vi "Local_Sense_Cmd_v1.vi"(7 "Control Board VISA":refnum<visa-resource-name>="ControlBoard", 8 "error in (no error)":errorcluster, 9 "Message IN":string, 10 "Relay Control":bool[](array[boolean]), 11 "LocalSenseRelayTask":refnum<k21>="BTS_LocalSenseRelays") -> (0 "error out":errorcluster, 1 "Message OUT":string, 2 "Voltage Array":dbl[](array[numeric]), 3 "LocalSenseRelayTaskOut":refnum<k21>)   [LabVIEW 2019]
uses:
  Ctls/ADC_Select_v1.ctl
  <vilib>/DAQmx/write.llb/DAQmx Write (Digital 1D Bool NChan 1Samp 1Line).vi
  <vilib>/DAQmx/miscellaneous.llb/DAQmx Fill In Error Info.vi
panel:
  out "Vline_ca":dbl
  out "Vline_ab":dbl
  out "Vline_bc":dbl
  out "Control Board OUT":refnum<visa-resource-name>
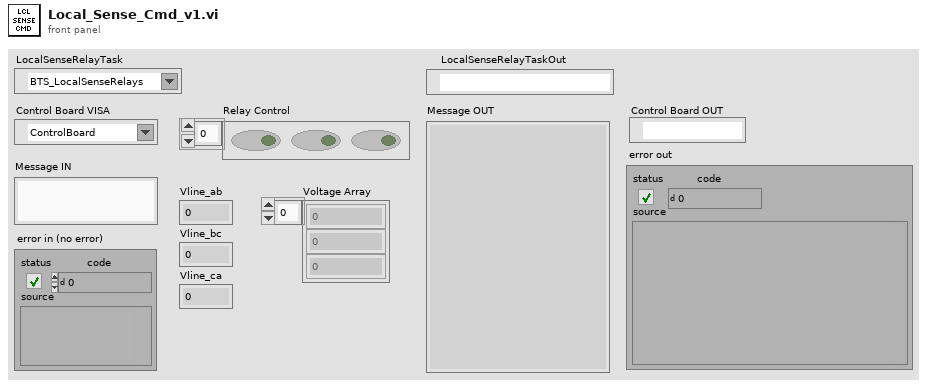
[diagram p1: front panel]
types:
  T1 = typedef "ADC_Select_v1.ctl" = enum16{"INVA_ISENSE_U", "INVA_ISENSE_V", "INVA_ISENSE_W", "INVA_UDC", "INVA_TEMP", "HB_TEMP", "AUXB_TEMP", "VLINE_AB", "VLINE_BC", "VLINE_CA", "VSENSE_POS_24V", "VSENSE_POS_5V", "VSENSE_NEG_15V", "INVB_ISENSE_U", "INV_B_ISENSEV", "INVB_ISENSE_W", "INVB_UDC", "INVB_TEMP", "AUXA_TEMP", "AUXC_TEMP", "VOUT_AB", "VOUT_BC", "VOUT_CA", "VSENSE_POS_15V", "VSENSE_POS_3P3V", "TEST_POINT"}
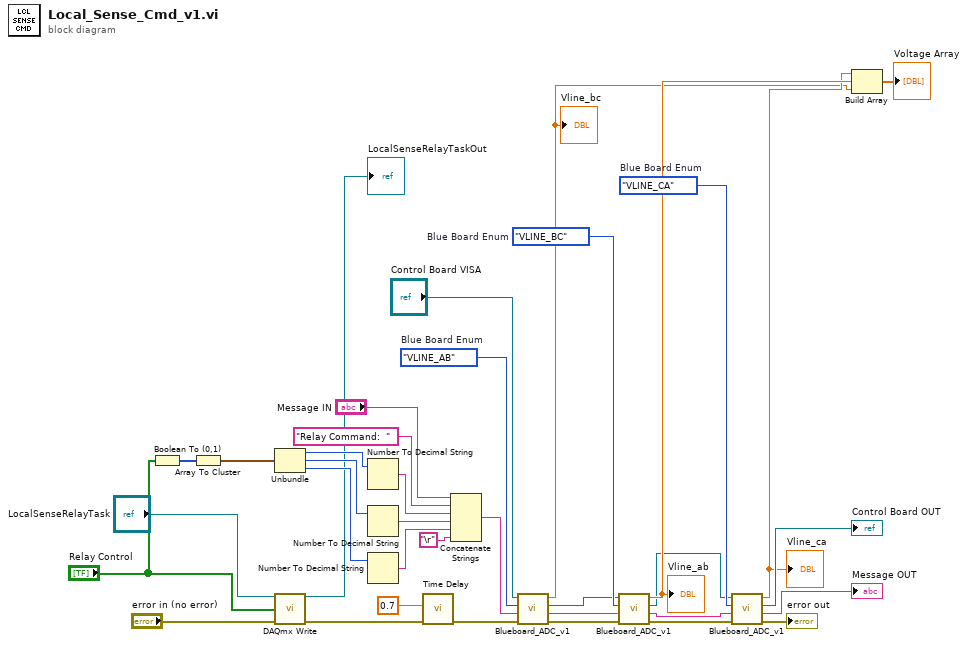
[diagram p0: block diagram]
diagram:
  w6 = ADC_Select_v1."VLINE_CA"  # Blue Board Enum
  w7 = ADC_Select_v1."VLINE_BC"  # Blue Board Enum
  w8 = ADC_Select_v1."VLINE_AB"  # Blue Board Enum
  n1 = Boolean To (0,1)(Boolean="Relay Control") -> (0, 1=w23:i16[])
  n2 = Array To Cluster(array=w23) -> (cluster=w22:cluster{"[0]":i16, "[1]":i16, "[2]":i16})
  n3 = Unbundle(w22) -> ("[0]"=w21:i16, "[1]"=w20:i16, "[2]"=w19:i16)
  n4 = call-poly <vilib>:"DAQmx Write.vi"("task/channels in"="LocalSenseRelayTask", "data"="Relay Control", "error in"="error in (no error)") -> ("task out"=→"LocalSenseRelayTaskOut":refnum<k21>, "error out"=w34:errorcluster)  [unwired: 10 in, 1 out]
  n5 = Number To Decimal String(number=w21) -> (decimal integer string=w16:string)  [unwired: 1 in]
  n6 = Number To Decimal String(number=w20) -> (decimal integer string=w17:string)  [unwired: 1 in]
  n7 = Number To Decimal String(number=w19) -> (decimal integer string=w18:string)  [unwired: 1 in]
  n8 = call "Time Delay"("error in (no error)"=w34, "Delay Time (s)"=0.7) -> ("error out"=w31:errorcluster)  [unwired: 9 in]
  n9 = Concatenate Strings("Message IN", "Relay Command:  ", w16, w17, w18, "\r") -> (w15:string)
  n10 = call "Blueboard_ADC_v1.vi"("error in (no error)"=w31, "Message IN"=w15, "Blue Board Enum"=w8, "ControlBoard VISA"="Control Board VISA") -> ("error out"=w36:errorcluster, "Message OUT"=w14:string, "VISA Refnum out"=w4:refnum<visa-resource-name>, "Result"=w28:dbl)  [unwired: 4 in]
  "Vline_bc" <- w28
  n11 = call "Blueboard_ADC_v1.vi"("error in (no error)"=w36, "Message IN"=w14, "Blue Board Enum"=w7, "ControlBoard VISA"=w4) -> ("error out"=w35:errorcluster, "Message OUT"=w13:string, "VISA Refnum out"=w3:refnum<visa-resource-name>, "Result"=w30:dbl)  [unwired: 4 in]
  "Vline_ab" <- w30
  n12 = call "Blueboard_ADC_v1.vi"("error in (no error)"=w35, "Message IN"=w13, "Blue Board Enum"=w6, "ControlBoard VISA"=w3) -> ("error out"=→"error out":errorcluster, "Message OUT"=→"Message OUT":string, "VISA Refnum out"=→"Control Board OUT":refnum<visa-resource-name>, "Result"=w29:dbl)  [unwired: 4 in]
  "Vline_ca" <- w29
  n13 = Build Array(w29, w30, w28) -> (→"Voltage Array":dbl[])
